vi "control_data.vi"(1 "待处理数据":u8[](array[numeric])) -> (0 "输出簇":T1)   [LabVIEW 2014]
panel:
  out "x*y 2":dbl
  out "x*y":dbl
  out "16位整型":u16
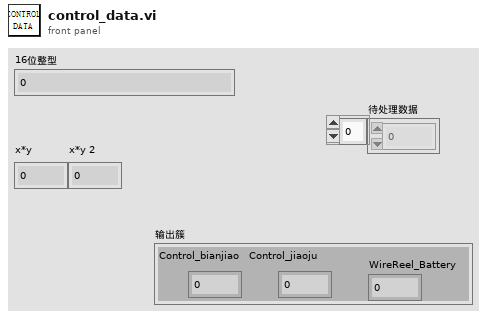
[diagram p1: front panel]
types:
  T1 = cluster{"Control_bianjiao":u8, "Control_jiaoju":u8, "WireReel_Battery":dbl}
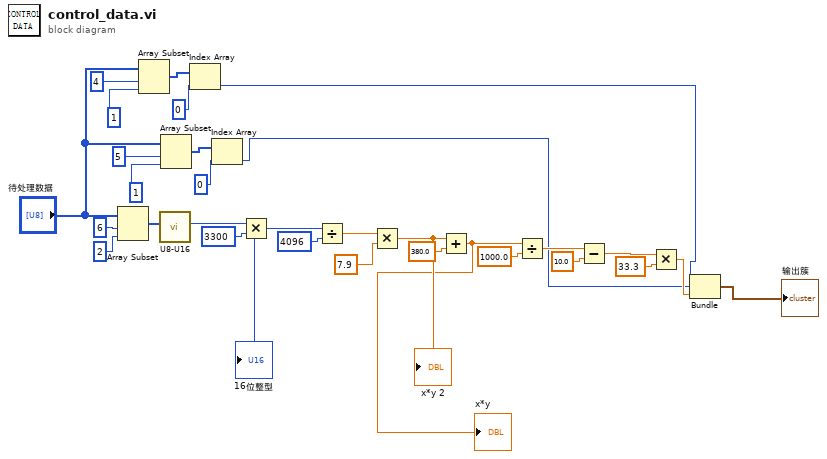
[diagram p0: block diagram]
diagram:
  n1 = Array Subset(array="待处理数据", index=6 ("索引"), length=2 ("索引")) -> (w14:u8[])
  n2 = Array Subset(array="待处理数据", index=4 ("长度（剩余）"), length=1 ("长度（剩余）")) -> (w10:u8[])
  n3 = call "U8-U16.vi"("数组"=w14) -> ("16位整型"=w29:u16)  [unwired: 8 in, 1 out]
  "16位整型" <- w29
  n4 = Array Subset(array="待处理数据", index=5 ("长度（剩余）"), length=1 ("长度（剩余）")) -> (w5:u8[])
  n5 = Index Array(array=w10, index=0 ("索引")) -> (element=w8:u8)
  n6 = Index Array(array=w5, index=0 ("索引")) -> (element=w1:u8)
  n7 = Multiply(x=w29, y=3300) -> (x*y=w26:i32)
  n8 = Divide(x=w26, y=4096) -> (x/y=w24:dbl)
  n9 = Multiply(x=w24, y=7.9) -> (x*y=w23:dbl)
  "x*y 2" <- w23
  n10 = Add(x=w23, y=380.0) -> (x+y=w11:dbl)
  "x*y" <- w11
  n11 = Divide(x=w11, y=1000.0) -> (x/y=w20:dbl)
  n12 = Subtract(x=w20, y=10.0) -> (x-y=w18:dbl)
  n13 = Multiply(x=w18, y=33.3) -> (x*y=w2:dbl)
  n14 = Bundle(w8, w1, w2) -> (→"输出簇":cluster{u8, u8, dbl})  [unwired: 1 in]
